vi "Delete Cache.vi"(8 "error in":errorcluster, 11 "IPath Getter.lvclass":refnum<class "IPath Getter.lvclass">) -> (0 "error out":errorcluster)   [LabVIEW 2020, in "Public API.lvlib"]
doc: "Deletes <b>Cache File</b> if it exists."
uses:
  Public API.lvlib
  <userlib>/_OpenG.lib/file/file.llb/openg_file.lvlib
  <userlib>/_OpenG.lib/file/file.llb/File Exists - Scalar__ogtk.vi
  IPath Getter/IPath Getter.lvclass
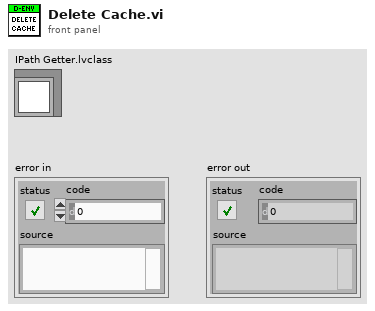
[diagram p1: front panel]
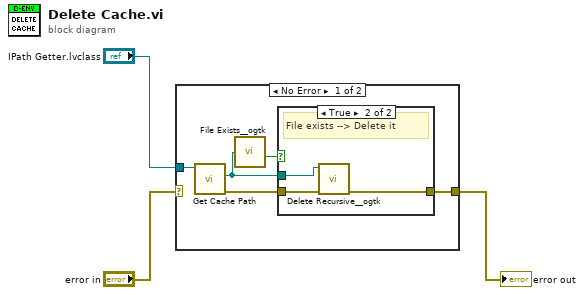
[diagram p0: block diagram]
diagram:
  n1 = case shown="No Error" "error in" {
    selector: "error in" -> [_ w13]
    tunnel: [w7 w13] -> w2
    tunnel: "IPath Getter.lvclass" -> [w5 _]
    frame No Error {
      n2 = call-dynamic "Get Cache Path.vi"("IPath Getter in"=w5) -> ("error out"=w8:errorcluster, "Path"=w4:path)  [unwired: 9 in]
      n3 = call-poly <userlib>:"File Exists__ogtk.vi"("file path"=w4) -> ("exists"=w6:bool)  [unwired: 6 in, 1 out]
      n4 = case shown="True" w6 {
        tunnel: w4 -> [_ w10]
        tunnel: w8 -> [w9 w12]
        tunnel: [w9 w11] -> w7
        frame False {
          # "File does not exist"
        }
        frame True {
          # "File exists --> Delete it"
          n5 = call <userlib>:"Delete Recursive__ogtk.vi"("error in (no error)"=w12, "Path"=w10) -> ("error out"=w11:errorcluster)  [unwired: 8 in, 1 out]
        }
      }
    }
    frame Error {
      # "Pass error without further action"
    }
  }
  "error out" <- w2
